vi "搜索数据.vi"(7 "condition":string, 8 "error in (no error)":errorcluster, 9 "database":string(combo)="database1.mdb") -> (0 "error out":errorcluster, 3 "data":string[][](array[string]))   [LabVIEW 2016]
uses:
  <vilib>/Utility/sysdir.llb/System Directory Type.ctl
  <vilib>/addons/database/Connection.llb/DB Tools Open Connec (String).vi
  <vilib>/addons/database/Connection.llb/Conn Execute.vi
  <vilib>/addons/database/Recordset.llb/Rec Fetch Recordset Data (R).vi
  <vilib>/addons/database/Recordset.llb/Rec Destroy - Connection.vi
  <vilib>/addons/database/_DB Variant To Data/Database Variant To Data.xnode
  <vilib>/addons/database/NI_Database_API.lvlib
panel:
  # "SELECT Format([时间],\"yyyy/mm/dd hh:00:00\") AS 按小时平均,Round(Avg([检测值]),3) as [检测平均值]\nFROM(select * from  where 测量模式 ='水样测试' and 数据类型 ='N' and 时间 >=#2021/05/05 02:02:02#and 时间 <=#2021/12/21 12:12:12#) \nGROUP BY Format([时间],\"yyyy/mm/dd hh:00:00\") order by Format([时间],\"yyyy/mm/dd hh:00:00\") asc;"
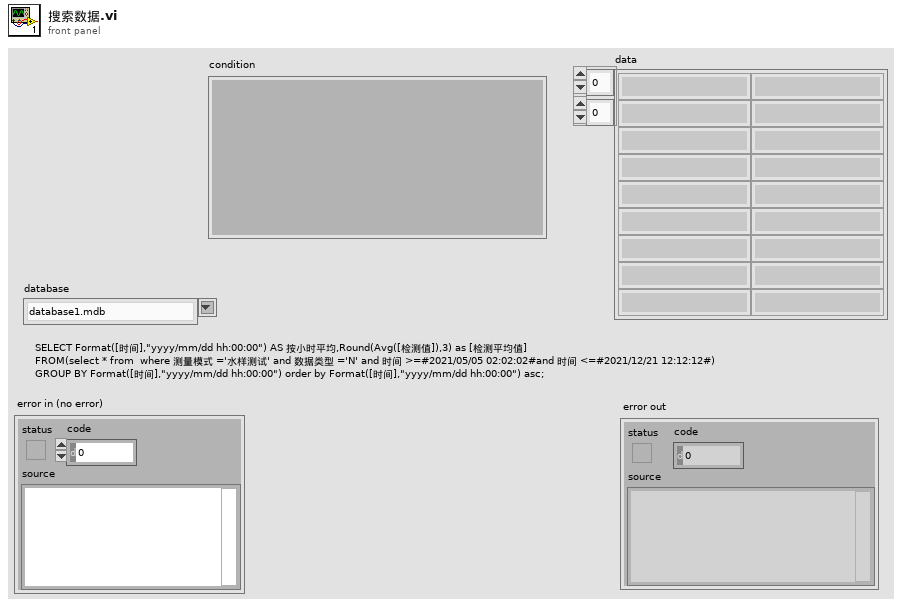
[diagram p1: front panel]
types:
  T1 = typedef "System Directory Type.ctl" = i32
  T2 = typedef "NI_Database_API.lvlib/Conn ObjectReference.ctl" = refnum<k1>
  T3 = typedef "NI_Database_API.lvlib/Rec ObjectReference.ctl" = refnum<k1>
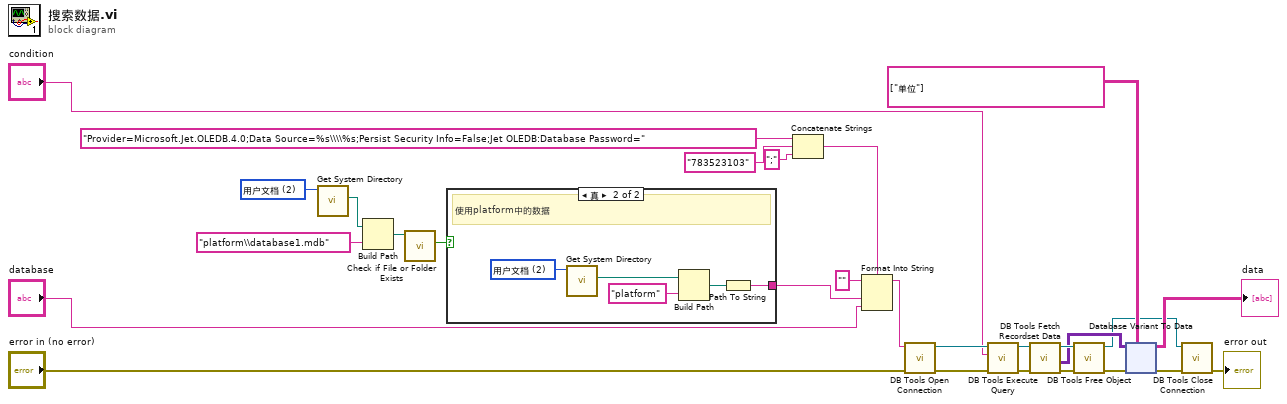
[diagram p0: block diagram]
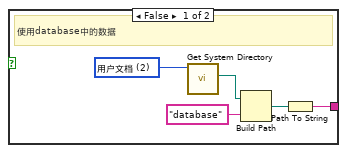
[diagram p2: hidden frame]
diagram:
  w22 = T1 2 items=["用户目录"=0, "用户桌面"=1, "用户文档"=2, "用户应用程序数据"=3, "用户设置"=4, "用户临时目录"=5, "公共文档"=6, "公共应用程序数据"=7, "公共设置"=8, "公共缓存"=13, "系统核心库"=9, "系统安装库"=10, "应用程序文件"=11, "启动盘根目录"=12] ("system directory type")
  n1 = call <vilib>:"Get System Directory.vi"("system directory type"=w22) -> ("system directory"=w23:path)  [unwired: 10 in]
  n2 = Build Path(base path=w23, name or relative path="platform\\database1.mdb" ("condition")) -> (appended path=w21:path)
  n3 = call <vilib>:"Check if File or Folder Exists.vi"("path"=w21) -> ("file or folder exists?"=w19:bool)  [unwired: 8 in, 2 out]
  n4 = case shown="真" w19 {
    tunnel: [w29 w34] -> w18
    frame False {
      w32 = T1 2 items=["用户目录"=0, "用户桌面"=1, "用户文档"=2, "用户应用程序数据"=3, "用户设置"=4, "用户临时目录"=5, "公共文档"=6, "公共应用程序数据"=7, "公共设置"=8, "公共缓存"=13, "系统核心库"=9, "系统安装库"=10, "应用程序文件"=11, "启动盘根目录"=12] ("system directory type")
      # "使用database中的数据"
      n5 = call <vilib>:"Get System Directory.vi"("system directory type"=w32) -> ("system directory"=w31:path)  [unwired: 10 in]
      n6 = Build Path(base path=w31, name or relative path="database" ("condition")) -> (appended path=w33:path)
      n7 = Path To String(path=w33) -> (string=w29:string)
    }
    frame True {
      w38 = T1 2 items=["用户目录"=0, "用户桌面"=1, "用户文档"=2, "用户应用程序数据"=3, "用户设置"=4, "用户临时目录"=5, "公共文档"=6, "公共应用程序数据"=7, "公共设置"=8, "公共缓存"=13, "系统核心库"=9, "系统安装库"=10, "应用程序文件"=11, "启动盘根目录"=12] ("system directory type")
      # "使用platform中的数据"
      n8 = call <vilib>:"Get System Directory.vi"("system directory type"=w38) -> ("system directory"=w37:path)  [unwired: 10 in]
      n9 = Build Path(base path=w37, name or relative path="platform" ("condition")) -> (appended path=w35:path)
      n10 = Path To String(path=w35) -> (string=w34:string)
    }
  }
  n11 = Concatenate Strings("Provider=Microsoft.Jet.OLEDB.4.0;Data Source=%s\\\\%s;Persist Security Info=False;Jet OLEDB:Database Password=" ("格式字符串"), "783523103" ("字符串"), ";" ("字符串")) -> (w24:string)
  n12 = Format Into String(format string=w24, initial string="" ("初始字符串"), w18, "database") -> (resulting string=w16:string)  [unwired: 1 in, 1 out]
  n13 = call-poly <vilib>:"DB Tools Open Connection.vi"("error in (no error)"="error in (no error)", "connection information"=w16) -> ("error out"=w7:errorcluster, "connection reference"=w8:T2)  [unwired: 6 in]
  n14 = call-poly <vilib>:"DB Tools Execute Query.vi"("error in (no error)"=w7, "SQL query"="condition", "connection reference"=w8) -> ("error out"=w9:errorcluster, "recordset reference"=w10:T3)  [unwired: 5 in]
  n15 = call-poly <vilib>:"DB Tools Fetch Recordset Data.vi"("error in (no error)"=w9, "recordset reference"=w10) -> ("error out"=w4:errorcluster, "recordset data"=w3:variant[][], "recordset reference out"=w5:T3)  [unwired: 3 in]
  n16 = call-poly <vilib>:"DB Tools Free Object.vi"("error in (no error)"=w4, "recordset reference"=w5) -> ("error out"=w2:errorcluster, "connection reference"=w1:T2)  [unwired: 8 in]
  n17 = xnode "Database Variant To Data"("database variant"=w3, "error in (no error)"=w2, "type"=string[][] [["单位"]]) -> ("data"=→"data":string[][], "error out"=w14:errorcluster)
  n18 = call <vilib>:"DB Tools Close Connection.vi"("error in (no error)"=w14, "connection reference"=w1) -> ("error out"=→"error out":errorcluster)  [unwired: 5 in]
